vi "construct.vi"(8 "error in (no error)":errorcluster, 9 "configuration name":string, 10 "load config file?":bool=TRUE, 11 "ScanModeDL090923Scaffold in":refnum<class "ImagingModeDL100901FlexTrajectory.lvclass">) -> (0 "error out":errorcluster, 3 "ScanModeDL090923Scaffold out":refnum<class "ImagingModeDL100901FlexTrajectory.lvclass">)   [LabVIEW 2010, in "ImagingModeDL100901FlexTrajectory.lvclass"]
uses:
  ImagingModeDL100901FlexTrajectory.lvclass
  ImagingModeDL091001Scaffold/ImagingModeDL091001Scaffold/ImagingModeDL091001Scaffold.lvclass
  Trajectory/GenericTrajectory/GenericTrajectory/GenericTrajectory.lvclass
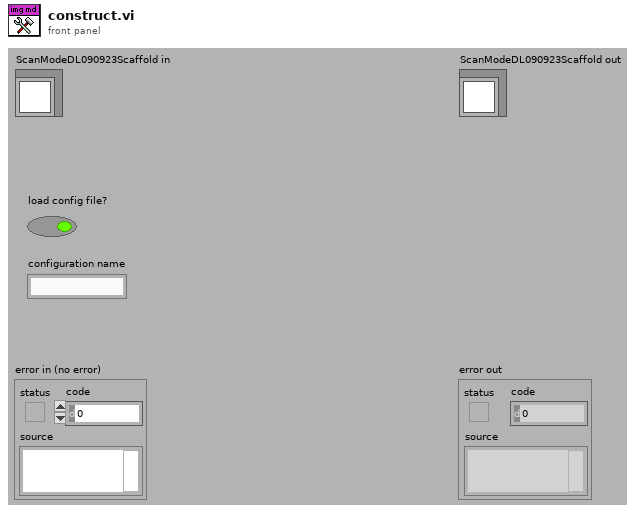
[diagram p1: front panel]
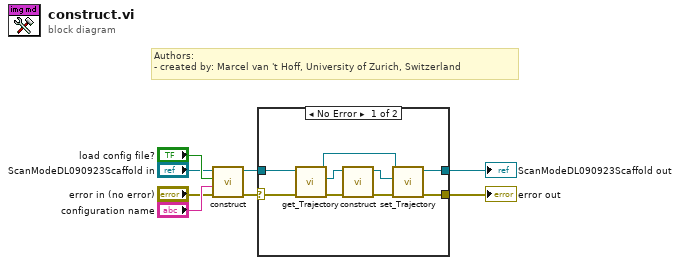
[diagram p0: block diagram]
diagram:
  # "Authors: \n- created by: Marcel van 't Hoff, University of Zurich, Switzerland"
  n1 = call-parent "construct.vi"("error in (no error)"="error in (no error)", "configuration name"="configuration name", "load config file?"="load config file?", "ScanModeDL090923Scaffold in"="ScanModeDL090923Scaffold in") -> ("error out"=w1:errorcluster, "ScanModeDL090923Scaffold out"=w2:refnum<class "ImagingModeDL100901FlexTrajectory.lvclass">)  [unwired: 6 in]
  n2 = case shown="No Error" w1 {
    selector: w1 -> [w9 w19]
    tunnel: [w17 w19] -> w5
    tunnel: [w16 w18] -> w4
    tunnel: w2 -> [w11 w18]
    frame No Error {
      n3 = call-dynamic "get_Trajectory.vi"("error in (no error)"=w9, "ScanModeDL090923Scaffold in"=w11) -> ("error out"=w13:errorcluster, "Trajectory"=w15:refnum<class "GenericTrajectory.lvclass">, "ScanModeDL090923Scaffold out"=w10:refnum<class "ImagingModeDL100901FlexTrajectory.lvclass">)  [unwired: 2 in, 5 out]
      n4 = call-dynamic "construct.vi"("error in (no error)"=w13, "GenericPlugin in"=w15) -> ("error out"=w12:errorcluster, "GenericPlugin out"=w14:refnum<class "GenericTrajectory.lvclass">)  [unwired: 8 in]
      n5 = call-dynamic "set_Trajectory.vi"("error in (no error)"=w12, "GenericTrajectory.lvclass"=w14, "ScanModeDL090923Scaffold in"=w10) -> ("error out"=w17:errorcluster, "ScanModeDL090923Scaffold out"=w16:refnum<class "ImagingModeDL100901FlexTrajectory.lvclass">)  [unwired: 7 in]
    }
    frame Error {
    }
  }
  "error out" <- w5
  "ScanModeDL090923Scaffold out" <- w4
